vi "Write Panels.vi"(8 "error in (no error)":errorcluster, 10 "Panels":T1(array[cluster]), 11 "Maui Manager in":refnum<class "Maui Manager.lvclass">) -> (0 "error out":errorcluster, 3 "Maui Manager out":refnum<class "Maui Manager.lvclass">)   [LabVIEW 2019, in "Maui Manager.lvclass"]
uses:
  Maui Manager.lvclass
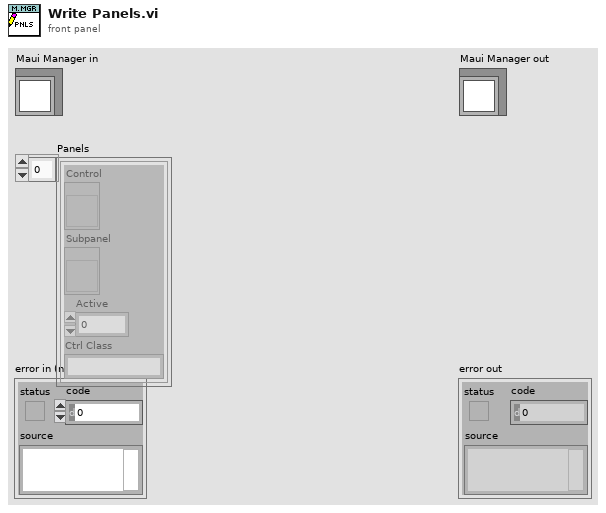
[diagram p1: front panel]
types:
  T1 = cluster{"Control":refnum<vi>, "Subpanel":refnum<vi>, "Active":i32, "Ctrl Class":string}[]
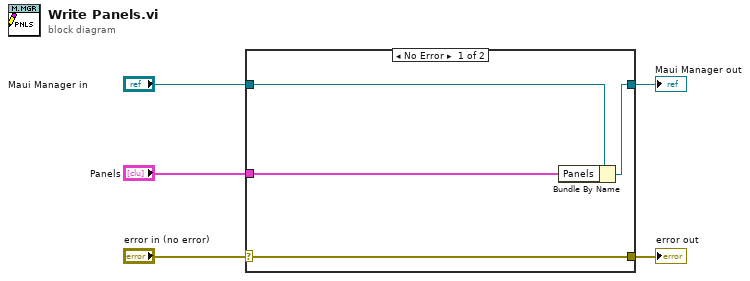
[diagram p0: block diagram]
diagram:
  n1 = case shown="No Error" "error in (no error)" {
    selector: "error in (no error)" -> [w9 w10]
    tunnel: [w9 w10] -> w4
    tunnel: [w7 w11] -> w2
    tunnel: "Maui Manager in" -> [w8 w11]
    tunnel: "Panels" -> [w6 _]
    frame No Error {
      n2 = Bundle By Name(cluster=w8, "Panels"=w6) -> (w7:refnum<class "Maui Manager.lvclass">)
    }
    frame Error {
    }
  }
  "error out" <- w4
  "Maui Manager out" <- w2
